vi "Write Result.vi"(0 "Scalar Path in":refnum<class "Scalar Path.lvclass">, 11 "error in (no error)":errorcluster) -> (4 "Scalar Path out":refnum<class "Scalar Path.lvclass">, 15 "error out":errorcluster)   [LabVIEW 2023, in "RFFixtureCharact.Public.lvlib" / "Scalar Path.lvclass"]
uses:
  Scalar Path.lvclass
  C:/srd-semi-rfcal-software/AuxTools/STSRFFixtureCharactUtility/Source/Code Modules/Common/Base Classes/Path/Path.lvclass
  Common/Result Accessor/Result Accessor.lvclass
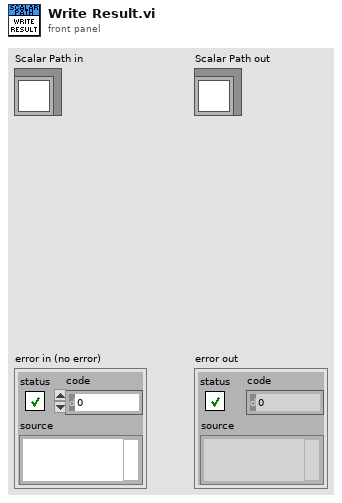
[diagram p1: front panel]
types:
  T1 = typedef "RFFixtureCharact.Public.lvlib/Scalar Path.lvclass/Scalar Charact Result.ctl" = cluster{"Port Power":dbl, "Reference Level":dbl, "Frequency":dbl, "Path Gain":dbl, "Out Of Limit":bool}
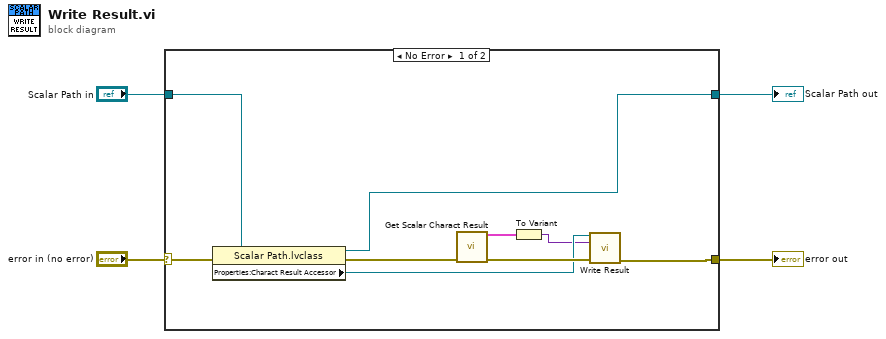
[diagram p0: block diagram]
diagram:
  n1 = case shown="No Error" "error in (no error)" {
    selector: "error in (no error)" -> [w13 w15]
    tunnel: "Scalar Path in" -> [w12 w14]
    tunnel: [w10 w14] -> w3
    tunnel: [w8 w15] -> w2
    frame No Error {
      n2 = property class="Scalar Path.lvclass"(reference=w12, error in=w13) -> (reference out=w10:refnum<class "Scalar Path.lvclass">, error out=w11:errorcluster, "Properties:Charact Result Accessor"=w7:refnum<class "Result Accessor.lvclass">)
      n3 = call "Get Scalar Charact Result.vi"("error in (no error)"=w11) -> ("Charact result"=w6:T1[], "error out"=w9:errorcluster)  [unwired: 13 in]
      n4 = To Variant(anything=w6) -> (Variant=w5:variant)
      n5 = call-dynamic "Write Result.vi"("Charact Result Accessor in"=w7, "Charact Result"=w5, "error in"=w9) -> ("error out"=w8:errorcluster)  [unwired: 11 in, 1 out]
    }
    frame Error {
    }
  }
  "error out" <- w2
  "Scalar Path out" <- w3
